vi "Rebin Histogram with Dialog.vi"(8 "error in (no error)":errorcluster, 11 "Original Bin Histogram":cluster{"Axis":dbl[], "Histogram":dbl[]}) -> (0 "error out":errorcluster, 1 "OK?":bool, 3 "Rebinned Histogram":cluster{"Axis":dbl[], "Histogram":dbl[]})   [LabVIEW 2019, in "Histogram Window.lvlib"]
uses:
  Histogram Window.lvlib
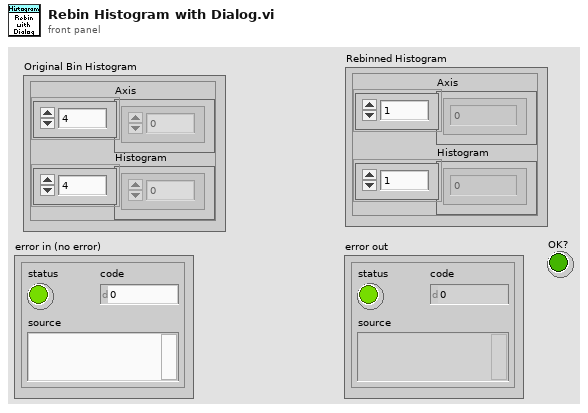
[diagram p1: front panel]
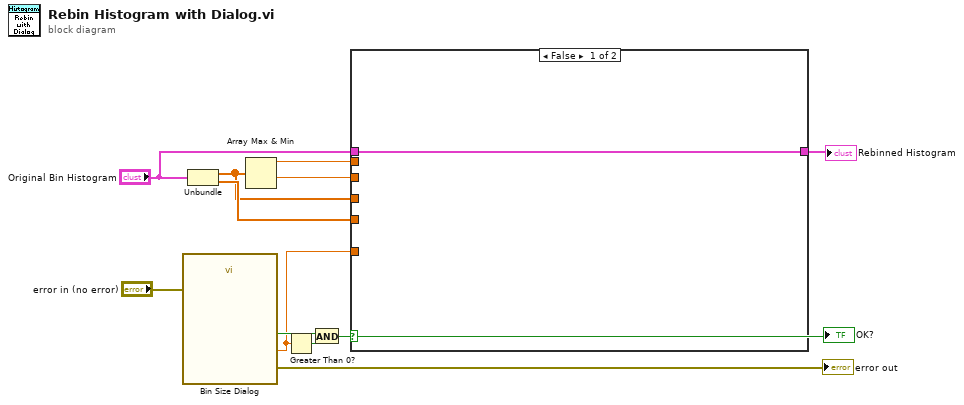
[diagram p0: block diagram]
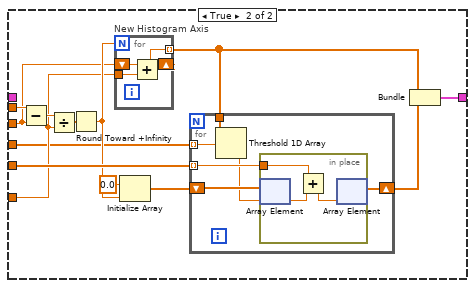
[diagram p2: hidden frame]
diagram:
  n1 = call "Bin Size Dialog.vi"("error in (no error)"="error in (no error)") -> ("Bin Size"=w5:dbl, "OK"=w10:bool, "error out"=→"error out":errorcluster)  [unwired: 16 in]
  n2 = Unbundle("Original Bin Histogram") -> ("Axis"=w3:dbl[], "Histogram"=w4:dbl[])
  n3 = Array Max & Min(array=w3) -> (max value=w7:dbl, min value=w6:dbl)  [unwired: 2 out]
  n4 = Greater Than 0?(x=w5) -> (x > 0?=w11:bool)
  n5 = And(x=w10, y=w11) -> (x .and. y?=w9:bool)
  "OK?" <- w9
  n6 = case shown="False" w9 {
    tunnel: w7 -> [_ w26]
    tunnel: w6 -> [_ w19]
    tunnel: w5 -> [_ w18]
    tunnel: w4 -> [_ w22]
    tunnel: w3 -> [_ w17]
    tunnel: [w13 w14] -> w2
    tunnel: "Original Bin Histogram" -> [w13 _]
    frame False {
    }
    frame True {
      n7 = Subtract(x=w26, y=w19) -> (x-y=w25:dbl)
      n8 = Divide(x=w25, y=w18) -> (x/y=w24:dbl)
      n9 = Round Toward +Infinity(x=w24) -> (ceil(x): smallest int >= x=w20:dbl)
      n10 = for "New Histogram Axis" {
        N: w20 -> [_]
        shift-right: [w28] -> _
        shift-left: w19 -> [w27]
        tunnel: w18 -> [w29]
        tunnel: [w27] -> w16 mode=indexing
        n11 = Add(x=w27, y=w29) -> (x+y=w28:dbl)
      }
      n12 = Initialize Array(0.0 ("element"), w20) -> (w21:dbl[])
      n13 = for {
        tunnel: w22 -> [w33] mode=indexing
        shift-right: [w34] -> w15
        shift-left: w21 -> [w35]
        tunnel: w17 -> [w31] mode=indexing
        tunnel: w16 -> [w32]
        n14 = Threshold 1D Array(2:w31, 3:w32) -> (0:w30:dbl)  [unwired: 1 in]
        n15 = in-place {
          in-place-border: w33 -> [w37]
          n16 = in-place-array #1(w35, w30) -> (w38:dbl)
          n17 = Add(x=w37, y=w38) -> (x+y=w36:dbl)
          n18 = in-place-array #1(w36) -> (w34:dbl[])  [unwired: 1 out]
        }
      }
      n19 = Bundle(w16, w15) -> (w14:cluster{dbl[], dbl[]})  [unwired: 1 in]
    }
  }
  "Rebinned Histogram" <- w2
